vi "Enable.vi"(0 "SystemEvents in":refnum<class "SystemEvents.lvclass">, 1 "event data":T1, 5 "error in (no error)":errorcluster) -> (14 "SystemEvents out":refnum<class "SystemEvents.lvclass">, 19 "error out":errorcluster)   [LabVIEW 2017, in "SystemEvents.lvclass"]
doc: "Fires the Enable event with the input parameters in attributes of the event data variant."
uses:
  SystemEvents.lvclass
  SystemEventData/EnableChangeEventData.ctl
  SystemEvents.lvclass/SystemEvents.ctl
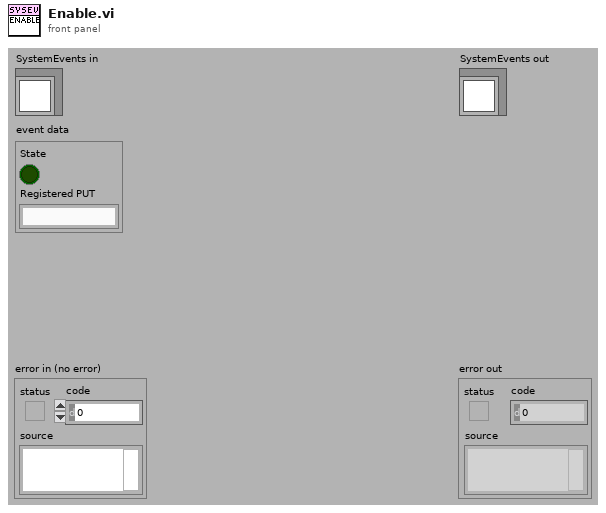
[diagram p1: front panel]
types:
  T1 = typedef "EnableChangeEventData.ctl" = cluster{"State":bool, "Registered PUT":string}
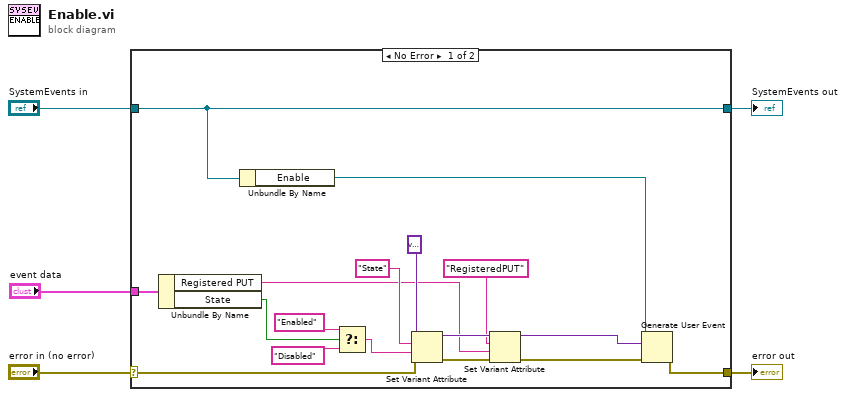
[diagram p0: block diagram]
diagram:
  n1 = case shown="No Error" "error in (no error)" {
    selector: "error in (no error)" -> [w8 w24]
    tunnel: [w21 w24] -> w4
    tunnel: [w22 w23] -> w2
    tunnel: "SystemEvents in" -> [w22 w23]
    tunnel: "event data" -> [w19 _]
    frame No Error {
      n2 = Unbundle By Name(w19) -> ("Registered PUT"=w11:string, "State"=w15:bool)
      n3 = Unbundle By Name(w22) -> ("Enable"=w20:refnum<user-event>)
      n4 = Select(t="Enabled" ("string"), s=w15, f="Disabled" ("string")) -> (s? t:f=w14:string)
      n5 = Set Variant Attribute(Variant=variant ("variant"), name="State", value=w14, error in=w8) -> (Variant out=w12:variant, error out=w9:errorcluster)  [unwired: 1 out]
      n6 = Set Variant Attribute(Variant=w12, name="RegisteredPUT", value=w11, error in=w9) -> (Variant out=w6:variant, error out=w7:errorcluster)  [unwired: 1 out]
      n7 = Generate User Event(user event=w20, event data cluster=w6, error in=w7) -> (error out=w21:errorcluster)  [unwired: 1 in, 1 out]
    }
    frame Error {
    }
  }
  "error out" <- w4
  "SystemEvents out" <- w2
